vi "connect.vi"(8 "error in (no error)":errorcluster, 11 "MB_TCP in":refnum<class "MB_TCP.lvclass">) -> (0 "error out":errorcluster, 3 "MB_TCP out":refnum<class "MB_TCP.lvclass">)   [LabVIEW 2021, in "MB_TCP.lvclass"]
uses:
  MB_TCP.lvclass
  MB_TCP.lvclass/MB_TCP.ctl
  NI_modbus_upd/TCP/TCP.lvclass/TCP.ctl
  NI_modbus_upd/TCP/TCP.lvclass
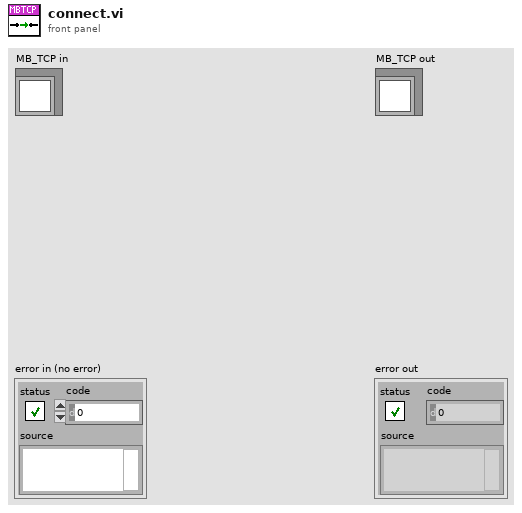
[diagram p1: front panel]
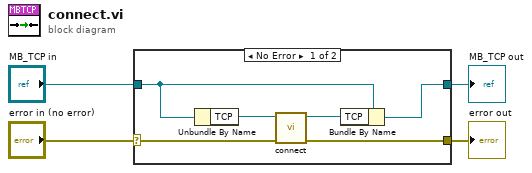
[diagram p0: block diagram]
diagram:
  n1 = case shown="No Error" "error in (no error)" {
    selector: "error in (no error)" -> [w9 w11]
    tunnel: [w5 w11] -> w3
    tunnel: [w6 w12] -> w1
    tunnel: "MB_TCP in" -> [w8 w12]
    frame No Error {
      n2 = Unbundle By Name(w8) -> ("TCP"=w10:refnum<class "TCP.lvclass">)
      n3 = call "connect.vi"("error in (no error)"=w9, "TCP in"=w10) -> ("error out"=w5:errorcluster, "TCP out"=w7:refnum<class "TCP.lvclass">)  [unwired: 8 in]
      n4 = Bundle By Name(cluster=w8, "TCP"=w7) -> (w6:refnum<class "MB_TCP.lvclass">)
    }
    frame Error {
    }
  }
  "error out" <- w3
  "MB_TCP out" <- w1
